vi "VI Tree.vi"   [LabVIEW 2023, in "Error Manager.lvlib" / "Log To File Loop Queue.lvclass"]
doc: "VI Tree\nThis VI lists all the public VIs and CTLs of the library."
uses:
  Log To File Loop Queue.lvclass
  Log To File Loop Queue.lvclass/Log To File Loop Queue.ctl
  Command (enum).ctl
panel:
  # "VI Tree\nSee the block diagram for the VI Tree"
types:
  T1 = typedef "Error Manager.lvlib/Log To File Loop Queue.lvclass/Command (enum).ctl" = enum16{"Init Loop", "Close Loop", "Log Error"}
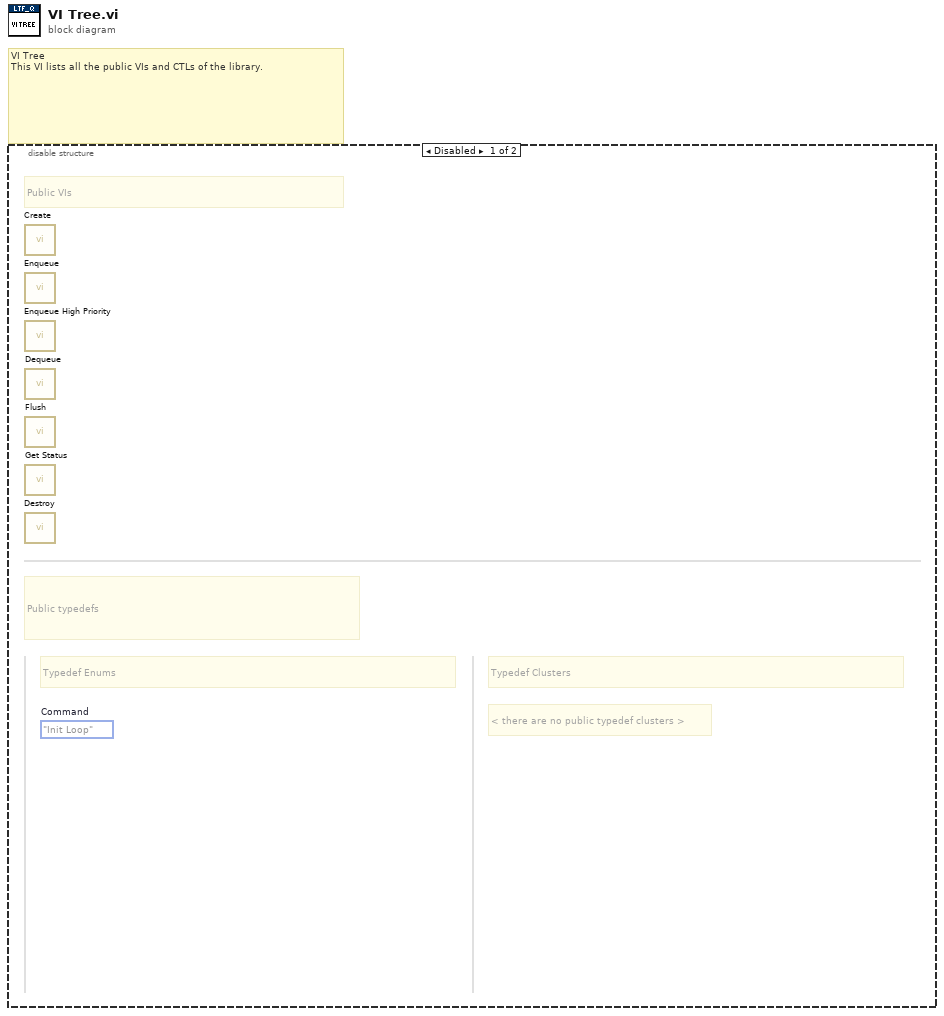
[diagram p0: block diagram]
diagram:
  # "VI Tree\nThis VI lists all the public VIs and CTLs of the library."
  n1 = disable-structure shown="Disabled" {
    frame Disabled {
      (unwired) Command_(enum)."Init Loop"  # Command
      # "< there are no public typedef clusters >"
      # "Typedef Clusters"
      # "Typedef Enums"
      # "Public typedefs"
      # "Public VIs"
      n2 = call "Create.vi"() -> ()  [unwired: 11 in, 1 out]
      n3 = call "Enqueue.vi"() -> ()  [unwired: 11 in, 1 out]
      n4 = call "Enqueue High Priority.vi"() -> ()  [unwired: 11 in, 1 out]
      n5 = call "Dequeue.vi"() -> ()  [unwired: 9 in, 3 out]
      n6 = call "Flush.vi"() -> ()  [unwired: 9 in, 3 out]
      n7 = call "Get Status.vi"() -> ()  [unwired: 9 in, 3 out]
      n8 = call "Destroy.vi"() -> ()  [unwired: 9 in, 3 out]
    }
    frame Enabled {
    }
  }
